vi "Set Awaited Event.vi"(8 "error in (no error)":errorcluster caption="entrée d'erreur (pas d'erreur)", 10 "Awaited Event":string, 11 "Class Event (Default) en entrée":refnum<class "Class Event (Default).lvclass">) -> (0 "error out":errorcluster caption="sortie d'erreur", 3 "Class Event (Default) en sortie":refnum<class "Class Event (Default).lvclass">)   [LabVIEW 2020, in "Library Instrument & Equipement.lvlib" / "Library Event.lvlib" / "Class Event (Default).lvclass"]
uses:
  Class Event (Default).lvclass
  Class Event (Default).lvclass/Class Event (Default).ctl
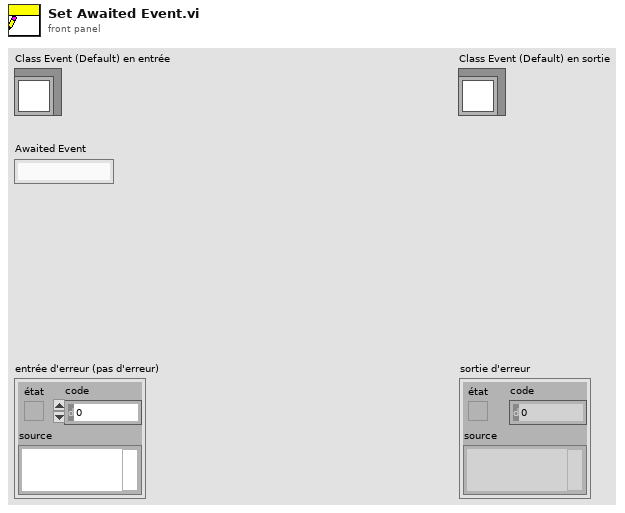
[diagram p1: front panel]
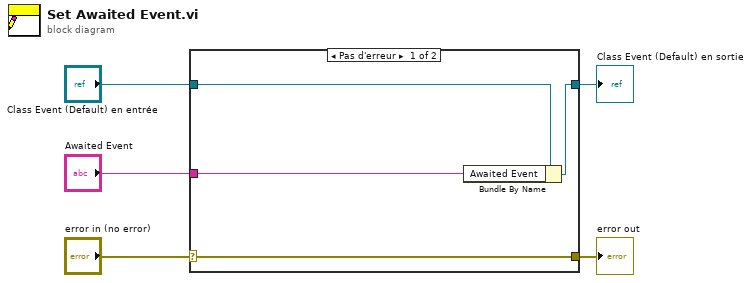
[diagram p0: block diagram]
diagram:
  n1 = case shown="Pas d'erreur" "error in (no error)" {
    selector: "error in (no error)" -> [w9 w10]
    tunnel: [w9 w10] -> w4
    tunnel: [w7 w11] -> w2
    tunnel: "Class Event (Default) en entrée" -> [w8 w11]
    tunnel: "Awaited Event" -> [w6 _]
    frame No Error {
      n2 = Bundle By Name(cluster=w8, "Awaited Event"=w6) -> (w7:refnum<class "Class Event (Default).lvclass">)
    }
    frame Error {
    }
  }
  "error out" <- w4
  "Class Event (Default) en sortie" <- w2
